vi "SeCrTS-DD AI config Divider.vi"(11 "AI config":T1(array[cluster])) -> (1 "AI C Pump":T1(array[cluster]), 2 "AI V Pump":T1(array[cluster]), 3 "AI  Storage":T1(array[cluster]))   [LabVIEW 2022 SP3]
panel:
  in  "Current card":string="PXI1Slot5"
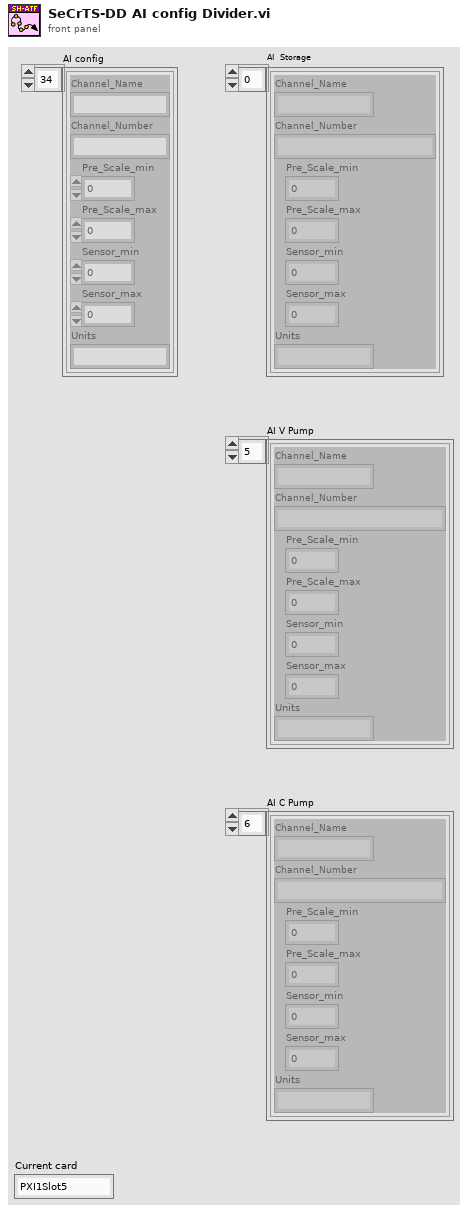
[diagram p1: front panel]
types:
  T1 = cluster{"Channel_Name":string, "Channel_Number":string, "Pre_Scale_min":dbl, "Pre_Scale_max":dbl, "Sensor_min":dbl, "Sensor_max":dbl, "Units":string}[]
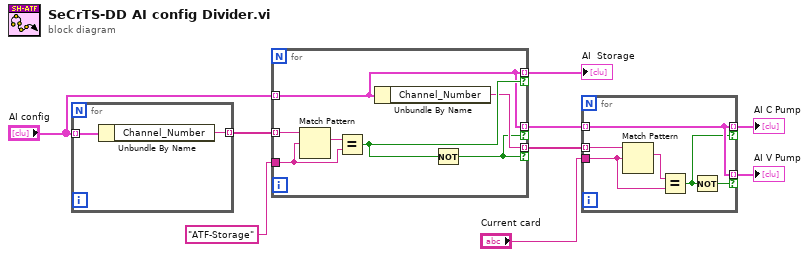
[diagram p0: block diagram]
diagram:
  n1 = for {
    tunnel: "AI config" -> [w11] mode=indexing
    tunnel: [w10] -> w6 mode=indexing
    n2 = Unbundle By Name(w11) -> ("Channel_Number"=w10:string)
  }
  n3 = for {
    tunnel: w6 -> [w16] mode=indexing
    tunnel: "ATF-Storage" ("C_DAQ Card") -> [w17]
    tunnel: [w14] -> w7 mode=indexing if=w15
    tunnel: "AI config" -> [w14] mode=indexing
    tunnel: [w14] -> w5 mode=indexing if=w12
    tunnel: [w13] -> w4 mode=indexing if=w12
    n4 = Match Pattern(string=w16, regular expression=w17) -> (match substring=w18:string)  [unwired: 1 in, 3 out]
    n5 = Equal?(x=w18, y=w17) -> (x = y?=w15:bool)
    n6 = Unbundle By Name(w14) -> ("Channel_Number"=w13:string)
    n7 = Not(x=w15) -> (.not. x?=w12:bool)
  }
  "AI  Storage" <- w7
  n8 = for {
    tunnel: w4 -> [w22] mode=indexing
    tunnel: "Current card" -> [w23]
    tunnel: [w21] -> w1 mode=indexing if=w20
    tunnel: w5 -> [w21] mode=indexing
    tunnel: [w21] -> w2 mode=indexing if=w19
    n9 = Match Pattern(string=w22, regular expression=w23) -> (match substring=w24:string)  [unwired: 1 in, 3 out]
    n10 = Equal?(x=w24, y=w23) -> (x = y?=w20:bool)
    n11 = Not(x=w20) -> (.not. x?=w19:bool)
  }
  "AI V Pump" <- w2
  "AI C Pump" <- w1
